vi "TopicSubset.vi"(8 "error in (no error)":errorcluster, 11 "Message Broker Interface TAP in":refnum<class "Message Broker Interface Ref.lvclass">) -> (0 "error out":errorcluster, 3 "Message Broker Interface TAP out":refnum<class "Message Broker Interface Ref.lvclass">)   [LabVIEW 2016, in "Stream Mediator.lvlib" / "Message Broker Interface Ref.lvclass"]
doc: "--\nCopyright © 2017 Composed SystemsI All rights reserved.\n\nAuthor: Jon McBee <jon.mcbee@composed.io>\n\nThis library is provided \"AS IS\" ,WITHOUT WARRANTIES OR\nCONDITIONS OF ANY KIND, either express or implied.\n\nComposed Systems -- composed.io\n\nStream 0.0.1.1\nJon McBee - Composed Systems\nCopyright (c) 2017, Composed Systems"
uses:
  <userlib>/Composed Systems/Stream/Mediator/Classes/Message Broker Interface Ref/Message Broker Interface Ref.lvclass
  <userlib>/Composed Systems/Stream/Mediator/Classes/Message Broker Interface Ref/Message Broker Interface Ref.lvclass/Message Broker Interface Ref.ctl
  <userlib>/Composed Systems/Stream/Mediator/Classes/Message Broker/Message Broker.lvclass
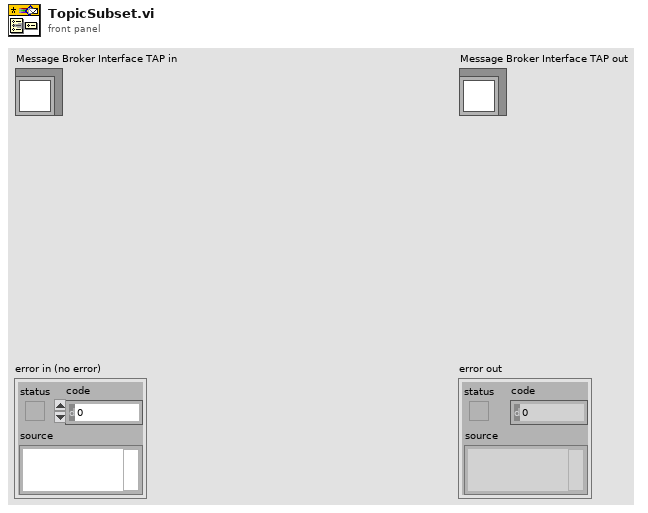
[diagram p1: front panel]
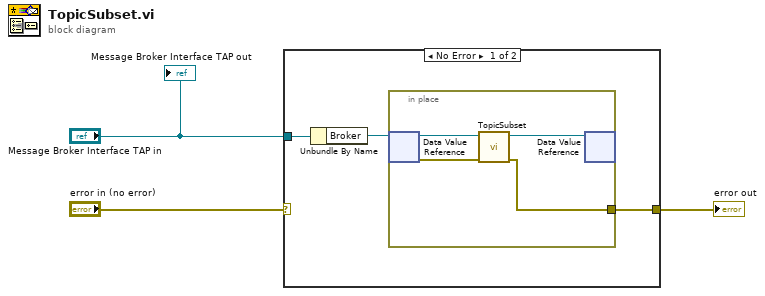
[diagram p0: block diagram]
diagram:
  n1 = case shown="No Error" "error in (no error)" {
    selector: "error in (no error)" -> [_ w11]
    tunnel: "Message Broker Interface TAP in" -> [w6 _]
    tunnel: [w4 w11] -> w1
    frame No Error {
      n2 = Unbundle By Name(w6) -> ("Broker"=w5:refnum<data-value>)
      n3 = in-place {
        in-place-border: [w7] -> w4
        n4 = in-place-dvr #1(w5) -> (w10:refnum<class "Message Broker.lvclass">, w8:errorcluster)
        n5 = call <userlib>:"TopicSubset.vi"("error in (no error)"=w8, "Message Broker in"=w10) -> ("error out"=w7:errorcluster, "Message Broker out"=w9:refnum<class "Message Broker.lvclass">)  [unwired: 8 in]
        n6 = in-place-dvr #1(w9) -> ()  [unwired: 2 out]
      }
    }
    frame Error {
    }
  }
  "error out" <- w1
  "Message Broker Interface TAP out" <- "Message Broker Interface TAP in"
